vi "AM Gen.vi"(7 "MIDI Waveform":waveform(dbl)[](graph), 9 "ModulationAmp":dbl=1.0 format="%0.2f", 10 "CarrierFre":dbl=0.0078125 format="%0.4e", 11 "CarrierAmp":dbl=1.0 format="%0.2f") -> (1 "FFTWave":cluster{"f0":dbl, "df":dbl, "magnitude":dbl[]}[](graph), 3 "输出簇":T1)   [LabVIEW 2018]
uses:
  <vilib>/measure/maspectr.llb/FFT Spectrum (Mag-Phase) for N Chan.vi
  <vilib>/measure/NI_MABase.lvlib
  <vilib>/measure/NI_MAPro.lvlib
panel:
  in  "簇":T1
  out "ModulationWave":waveform(dbl)[](graph)
  out "AM Output":waveform(dbl)[](graph)
  out "CarrieWave":waveform(dbl)(graph)
  in  "ModulationFre":dbl=0.0078125 format="%0.4e"
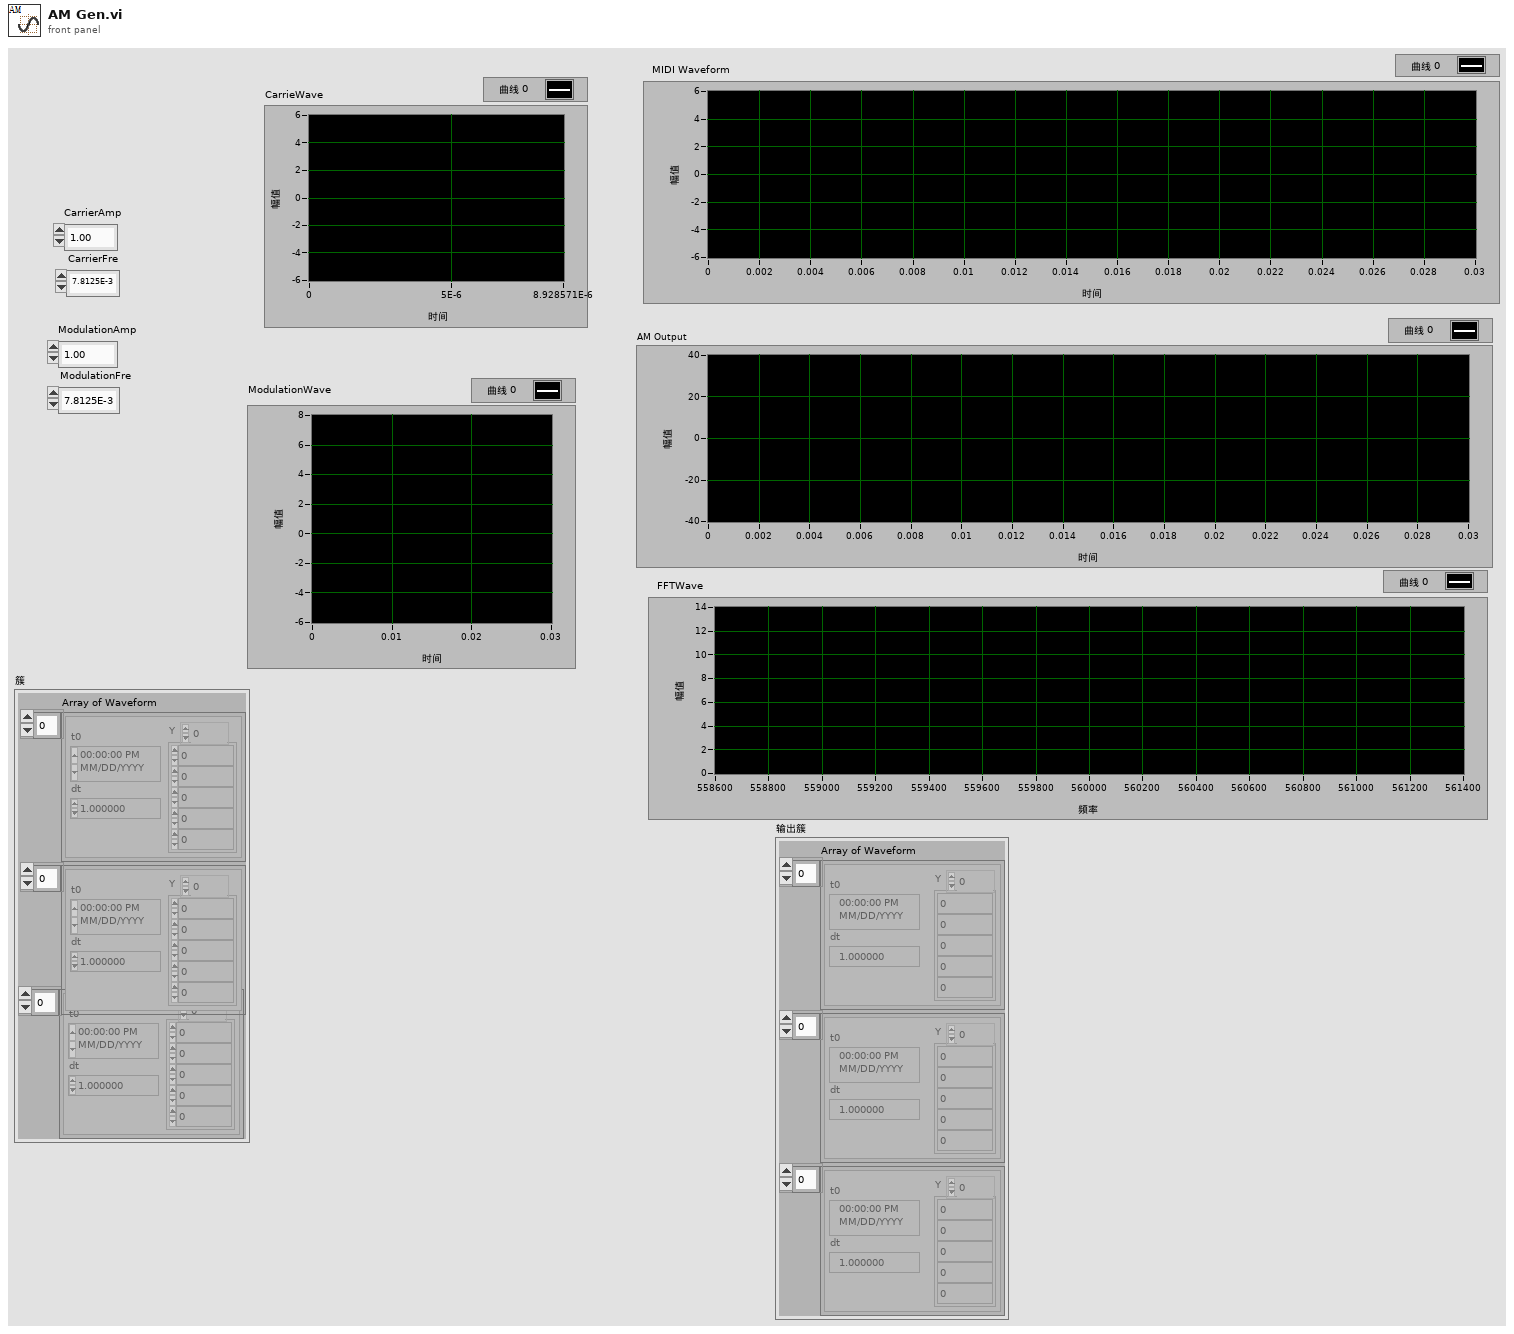
[diagram p1: front panel]
types:
  T1 = cluster{"Array of Waveform":waveform(dbl)[], waveform(dbl)[], waveform(dbl)[]}
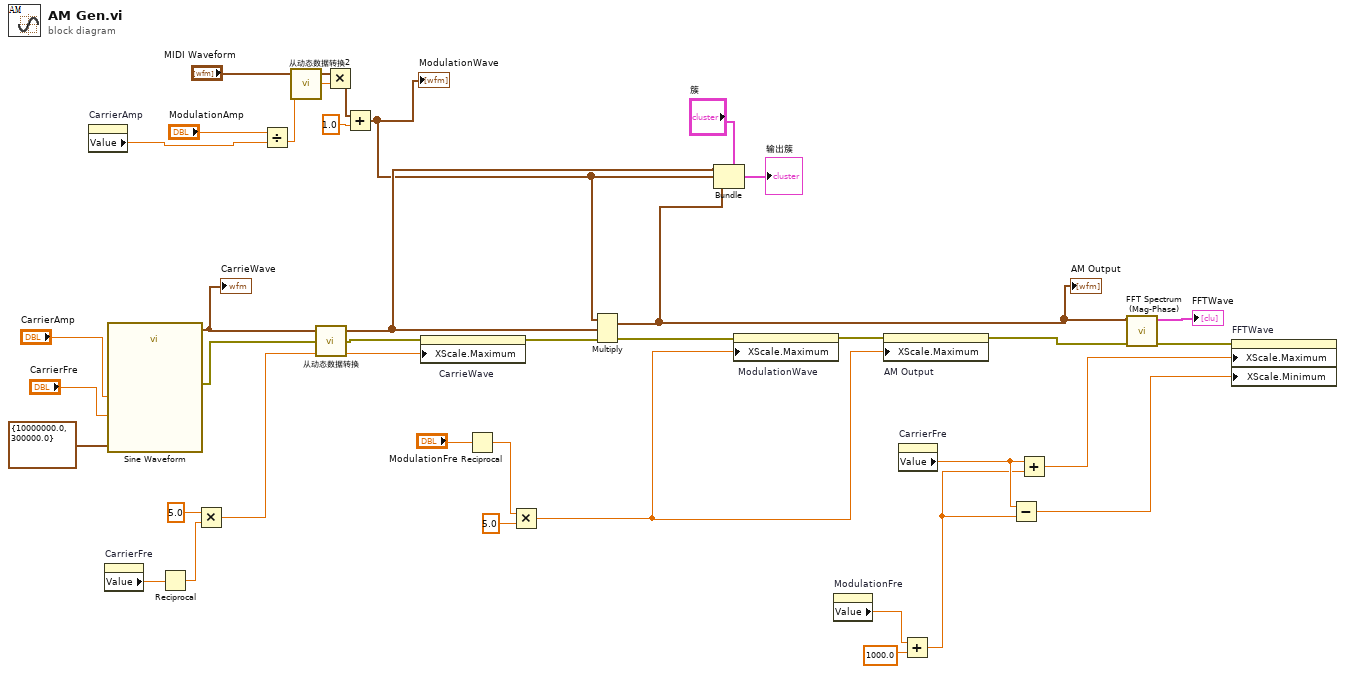
[diagram p0: block diagram]
diagram:
  n1 = property on="CarrierAmp" class="DigNum (严格)"() -> ("Value"=w5:dbl)  [unwired: 2 in, 2 out]
  n2 = property on="CarrierFre" class="DigNum (严格)"() -> ("Value"=w22:dbl)  [unwired: 2 in, 2 out]
  n3 = call <vilib>:"Sine Waveform.vi"("sampling info"=cluster{"Fs":dbl, "#s":dbl} {"Fs"=10000000.0, "#s"=300000.0}, "amplitude"="CarrierAmp", "frequency"="CarrierFre") -> ("error out"=w21:errorcluster, "signal out"=w37:waveform(dbl))  [unwired: 7 in]
  "CarrieWave" <- w37
  n4 = Reciprocal(x=w22) -> (1/x=w30:dbl)
  n5 = Multiply(x=5.0, y=w30) -> (x*y=w20:dbl)
  n6 = Divide(x="ModulationAmp", y=w5) -> (x/y=w35:dbl)
  n7 = call "从动态数据转换2"("Dynamic Data Type"="MIDI Waveform") -> ("Array of Waveform"=w4:waveform(dbl)[])  [unwired: 3 in]
  n8 = call "从动态数据转换"("Dynamic Data Type"=w37) -> ("Array of Waveform"=w12:waveform(dbl)[])  [unwired: 3 in]
  n9 = Multiply(x=w4, y=w35) -> (x*y=w34:waveform(dbl)[])
  n10 = Add(x=w34, y=1.0) -> (x+y=w11:waveform(dbl)[])
  "ModulationWave" <- w11
  n11 = property on="CarrieWave" class="WFGraph (严格)"(error in=w21, "XScale.Maximum"=w20) -> (error out=w29:errorcluster)  [unwired: 1 in, 1 out]
  n12 = Reciprocal(x="ModulationFre") -> (1/x=w26:dbl)
  n13 = Multiply(x=w26, y=5.0) -> (x*y=w25:dbl)
  n14 = Multiply(1:w12, 2:w11, 4:w29) -> (0:w10:waveform(dbl)[], 3:w28:errorcluster)
  "AM Output" <- w10
  n15 = Bundle(cluster="簇", "Array of Waveform"=w12, w11, w10) -> (→"输出簇":T1)
  n16 = property on="ModulationWave" class="WFGraph (严格)"(error in=w28, "XScale.Maximum"=w25) -> (error out=w27:errorcluster)  [unwired: 1 in, 1 out]
  n17 = property on="ModulationFre" class="DigNum (严格)"() -> ("Value"=w17:dbl)  [unwired: 2 in, 2 out]
  n18 = property on="AM Output" class="WFGraph (严格)"(error in=w27, "XScale.Maximum"=w25) -> (error out=w24:errorcluster)  [unwired: 1 in, 1 out]
  n19 = property on="CarrierFre" class="DigNum (严格)"() -> ("Value"=w16:dbl)  [unwired: 2 in, 2 out]
  n20 = Add(x=w17, y=1000.0) -> (x+y=w15:dbl)
  n21 = Subtract(x=w16, y=w15) -> (x-y=w13:dbl)
  n22 = Add(x=w16, y=w15) -> (x+y=w14:dbl)
  n23 = call-poly <vilib>:"FFT Spectrum (Mag-Phase).vi"("error in (no error)"=w24, "time signals"=w10) -> ("error out"=w19:errorcluster, "magnitudes"=→"FFTWave":cluster{"f0":dbl, "df":dbl, "magnitude":dbl[]}[])  [unwired: 5 in, 3 out]
  n24 = property on="FFTWave" class="WFGraph (严格)"(error in=w19, "XScale.Maximum"=w14, "XScale.Minimum"=w13) -> ()  [unwired: 1 in, 2 out]
